vi "Temps and MCs.vi"(8 "error in (no error)":errorcluster, 9 "Motor":i16, 11 "data":waveform(dbl)[](array[waveform])) -> (0 "error out":errorcluster, 1 "Numeric":dbl, 2 "DC value 3":dbl, 4 "DC value 2":dbl, 5 "DC value":dbl, 7 "Numeric 2":dbl)   [LabVIEW 2011]
uses:
  <vilib>/measure/madcrms.llb/Basic Averaged DC-RMS for 1 Chan.vi
  <vilib>/measure/NI_MAPro.lvlib
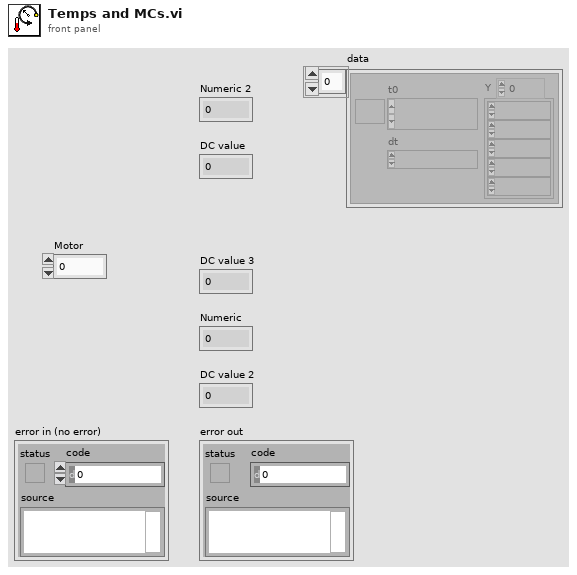
[diagram p1: front panel]
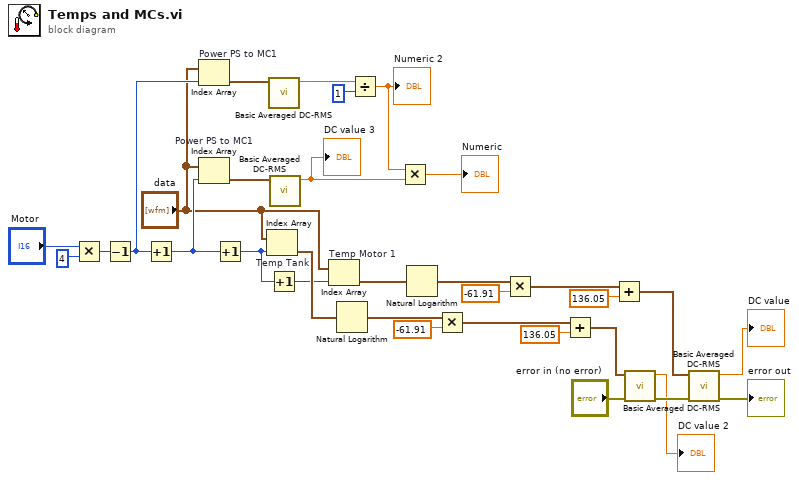
[diagram p0: block diagram]
diagram:
  n1 = Multiply(x="Motor", y=i16 4) -> (x*y=w9:i16)
  n2 = Decrement(x=w9) -> (x-1=w3:i16)
  n3 = Increment(x=w3) -> (x+1=w4:i16)
  n4 = Index Array "Power PS to MC1"(array="data", index=w3) -> (element=w22:waveform(dbl))
  n5 = Index Array "Power PS to MC1"(array="data", index=w4) -> (element=w24:waveform(dbl))
  n6 = Increment(x=w4) -> (x+1=w5:i16)
  n7 = Index Array "Temp Tank"(array="data", index=w5) -> (element=w26:waveform(dbl))
  n8 = call-poly <vilib>:"Basic Averaged DC-RMS.vi"("signal in"=w22) -> ("DC value"=w23:dbl)  [unwired: 7 in, 3 out]
  n9 = Increment(x=w5) -> (x+1=w6:i16)
  n10 = call-poly <vilib>:"Basic Averaged DC-RMS.vi"("signal in"=w24) -> ("DC value"=w25:dbl)  [unwired: 7 in, 3 out]
  "DC value 3" <- w25
  n11 = Index Array "Temp Motor 1"(array="data", index=w6) -> (element=w15:waveform(dbl))
  n12 = Natural Logarithm(1:w26) -> (0:w16:waveform(dbl))
  n13 = Divide(x=w23, y=1) -> (x/y=w20:dbl)
  "Numeric 2" <- w20
  n14 = Multiply(x=w20, y=w25) -> (x*y=→"Numeric":dbl)
  n15 = Natural Logarithm(1:w15) -> (0:w11:waveform(dbl))
  n16 = Multiply(x=w16, y=-61.91) -> (x*y=w18:waveform(dbl))
  n17 = Multiply(x=w11, y=-61.91) -> (x*y=w13:waveform(dbl))
  n18 = Add(x=w18, y=136.05) -> (x+y=w28:waveform(dbl))
  n19 = Add(x=w13, y=136.05) -> (x+y=w29:waveform(dbl))
  n20 = call-poly <vilib>:"Basic Averaged DC-RMS.vi"("error in (no error)"="error in (no error)", "signal in"=w28) -> ("error out"=w31:errorcluster, "DC value"=→"DC value 2":dbl)  [unwired: 6 in, 2 out]
  n21 = call-poly <vilib>:"Basic Averaged DC-RMS.vi"("error in (no error)"=w31, "signal in"=w29) -> ("error out"=→"error out":errorcluster, "DC value"=→"DC value":dbl)  [unwired: 6 in, 2 out]
